vi "FileIO-Update Parameter File Presets.vi"(0 "Presets":refnum<vi>, 7 "folder":path, 11 "selected":path) -> ()   [LabVIEW 2020]
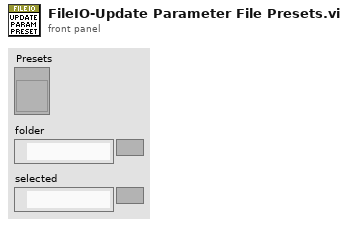
[diagram p1: front panel]
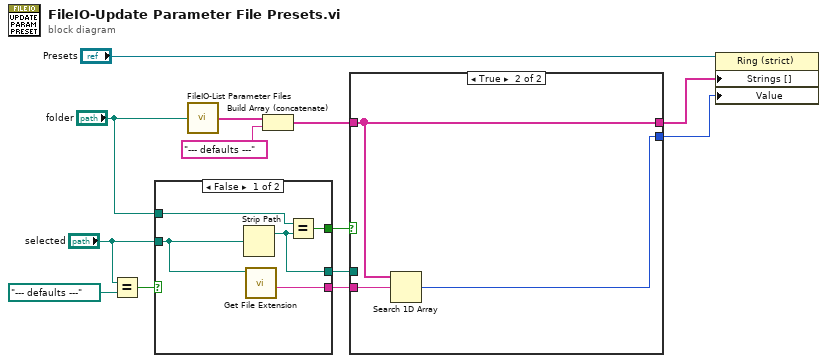
[diagram p0: block diagram]
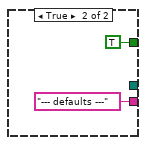
[diagram p2: hidden frame]
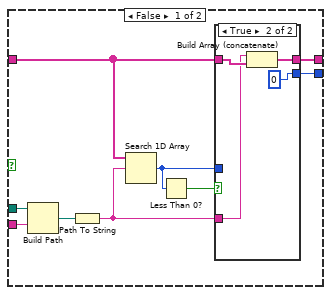
[diagram p3: hidden frame]
diagram:
  n1 = Equal?(x="selected", y=path "--- defaults ---") -> (x = y?=w5:bool)
  n2 = case shown="False" w5 {
    tunnel: "folder" -> [w18 _]
    tunnel: [w17 TRUE] -> w11
    tunnel: [w16 "--- defaults ---" ("filename without extension")] -> w10
    tunnel: "selected" -> [w15 _]
    tunnel: [w14 _] -> w4
    frame False {
      n3 = Strip Path(path=w15) -> (stripped path=w14:path)  [unwired: 1 out]
      n4 = call <vilib>:"Get File Extension.vi"("file"=w15) -> ("filename without extension"=w16:string)  [unwired: 6 in, 4 out]
      n5 = Equal?(x=w18, y=w14) -> (x = y?=w17:bool)
    }
    frame True {
    }
  }
  n6 = call "FileIO-List Parameter Files.vi"("folder"="folder") -> ("Parameter file names"=w12:string[])  [unwired: 14 in]
  n7 = Build Array (concatenate)(w12, "--- defaults ---") -> (w9:string[])
  n8 = case shown="True" w11 {
    tunnel: w9 -> [w24 w37]
    tunnel: w10 -> [w28 w38]
    tunnel: w4 -> [w29 _]
    tunnel: [w23 w37] -> w2
    tunnel: [w22 w36] -> w1
    frame False {
      n9 = Build Path(base path=w29, name or relative path=w28) -> (appended path=w27:path)
      n10 = Path To String(path=w27) -> (string=w21:string)
      n11 = Search 1D Array(1D array=w24, element=w21) -> (index of element=w25:i32)  [unwired: 1 in]
      n12 = Less Than 0?(x=w25) -> (x < 0?=w26:bool)
      n13 = case shown="True" w26 {
        tunnel: w25 -> [w30 _]
        tunnel: w24 -> [w31 w34]
        tunnel: [w31 w35] -> w23
        tunnel: [w30 0] -> w22
        tunnel: w21 -> [_ w33]
        frame False {
        }
        frame True {
          n14 = Build Array (concatenate)(w33, w34) -> (w35:string[])
        }
      }
    }
    frame True {
      n15 = Search 1D Array(1D array=w37, element=w38) -> (index of element=w36:i32)  [unwired: 1 in]
    }
  }
  n16 = property class="Ring (strict)"(reference="Presets", "Strings []"=w2, "Value"=w1) -> ()  [unwired: 1 in, 2 out]
